vi "GrabAllData.vi"(3 "Type of scan":u16, 4 "All files":string[](array[string]), 5 "error in":errorcluster, 6 "lines per plane mod":i32, 7 "Synth App?":bool, 8 "save?":bool=TRUE, 9 "Xmit Ring":i16, 10 "Start Record":i32, 11 "Reverse ?":bool) -> ()   [LabVIEW 2022 SP3]
uses:
  ScanningControl/Motion Controllers/-MotionRoutines/MotionGlobals.vi
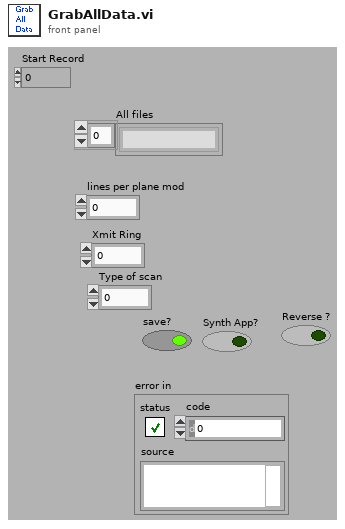
[diagram p1: front panel]
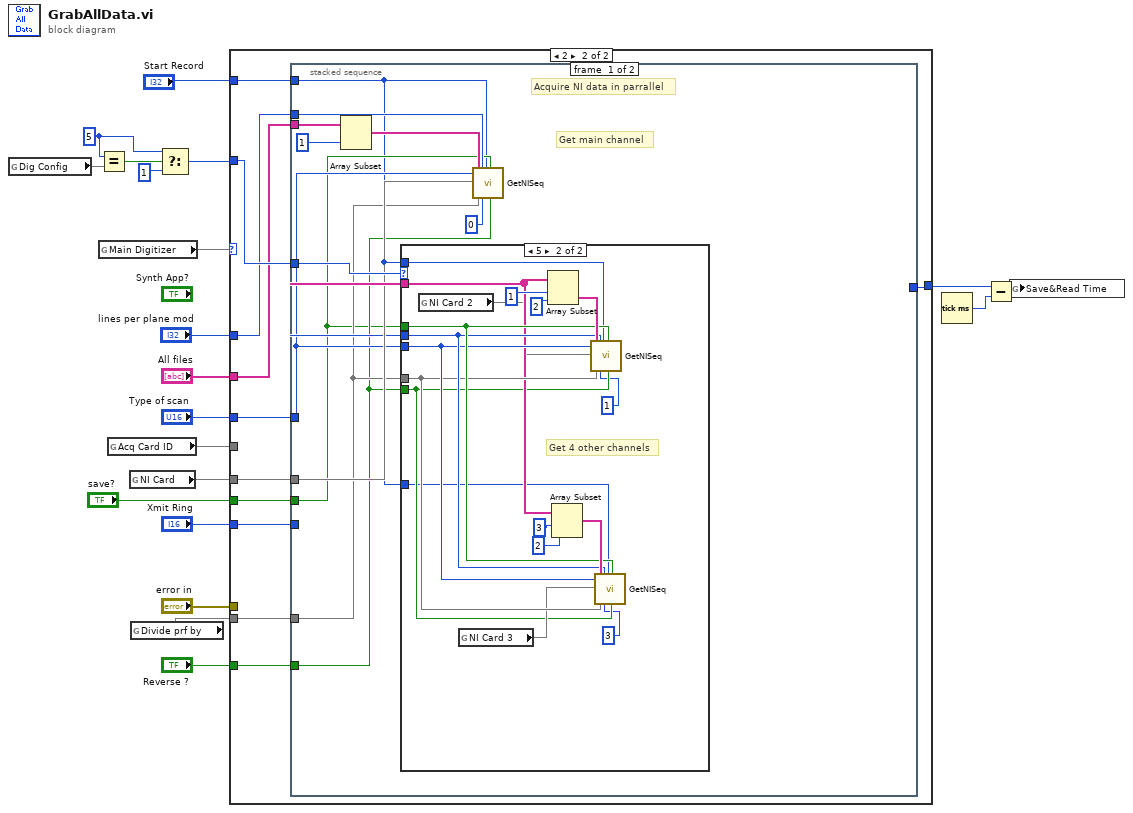
[diagram p0: block diagram]
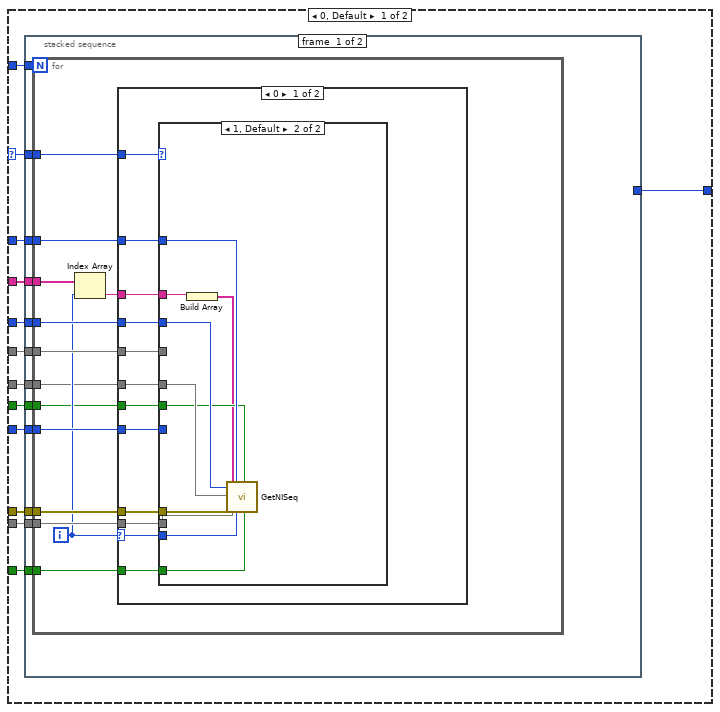
[diagram p2: hidden frame]
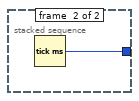
[diagram p5: hidden frame]
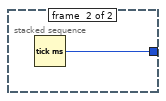
[diagram p7: hidden frame]
diagram:
  w20 = 5
  n1 = global read "MotionGlobals.vi" "Dig Config"() -> (w8)
  n2 = Equal?(x=w20, y=w8) -> (x = y?=w19:bool)
  n3 = global read "MotionGlobals.vi" "Main Digitizer"() -> (w5)
  n4 = global read "MotionGlobals.vi" "Acq Card ID"() -> (w10)
  n5 = global read "MotionGlobals.vi" "NI Card"() -> (w9)
  n6 = global read "MotionGlobals.vi" "Divide prf by"() -> (w7)
  n7 = Select(t=w20, s=w19, f=1) -> (s? t:f=w17:i32)
  n8 = case shown="2" w5 {
    selector: w5 -> [w22 _]
    tunnel: "All files" -> [w33 w91]
    tunnel: w17 -> [w32 w92]
    tunnel: "Xmit Ring" -> [w31 w87]
    tunnel: "Type of scan" -> [w30 w88]
    tunnel: "Reverse ?" -> [w29 w85]
    tunnel: "lines per plane mod" -> [w28 w89]
    tunnel: "error in" -> [w27 _]
    tunnel: w10 -> [w26 _]
    tunnel: w9 -> [w25 w90]
    tunnel: w7 -> [w24 w86]
    tunnel: "save?" -> [w23 w84]
    tunnel: [w21 w83] -> w4
    tunnel: "Start Record" -> [_ w82]
    frame 0, Default {
      n9 = stacked-sequence {
        tunnel: w33 -> [w45 _]
        tunnel: w32 -> [w44 _]
        tunnel: w31 -> [w43 _]
        tunnel: w30 -> [w42 _]
        tunnel: w29 -> [w41 _]
        tunnel: w28 -> [w40 _]
        tunnel: w27 -> [w39 _]
        tunnel: w26 -> [w38 _]
        tunnel: w25 -> [w37 _]
        tunnel: w24 -> [w36 _]
        tunnel: w23 -> [w35 _]
        tunnel: w22 -> [w34 _]
        tunnel: [_ w81] -> w21
        frame #0 {
          n10 = for {
            N: w44 -> [_]
            tunnel: w36 -> [w58]
            tunnel: w39 -> [w57]
            tunnel: w40 -> [w56]
            tunnel: w41 -> [w55]
            tunnel: w42 -> [w54]
            tunnel: w43 -> [w53]
            tunnel: w38 -> [w52]
            tunnel: w45 -> [w49]
            tunnel: w34 -> [w48]
            tunnel: w37 -> [w47]
            tunnel: w35 -> [w46]
            i -> [w50]
            n11 = Index Array(array=w49, index=w50) -> (element=w51:string)
            n12 = case shown="0" w50 {
              selector: w50 -> [w60 _]
              tunnel: w58 -> [w70 _]
              tunnel: w57 -> [w69 _]
              tunnel: w56 -> [w68 _]
              tunnel: w55 -> [w67 _]
              tunnel: w54 -> [w66 _]
              tunnel: w53 -> [w61 _]
              tunnel: w52 -> [w65 _]
              tunnel: w51 -> [w64 _]
              tunnel: w48 -> [w63 _]
              tunnel: w47 -> [w62 _]
              tunnel: w46 -> [w59 _]
              frame 0 {
                n13 = case shown="1, Default" w63 {
                  tunnel: w70 -> [_ w80]
                  tunnel: w69 -> [_ w79]
                  tunnel: w68 -> [_ w76]
                  tunnel: w67 -> [_ w75]
                  tunnel: w66 -> [_ w78]
                  tunnel: w61 -> [_ _]
                  tunnel: w65 -> [_ _]
                  tunnel: w64 -> [_ w73]
                  tunnel: w62 -> [_ w77]
                  tunnel: w60 -> [_ w71]
                  tunnel: w59 -> [_ w74]
                  frame 0 {
                    # "Get single channel Acqiris data"
                  }
                  frame 1, Default {
                    n14 = Build Array(w73) -> (w72:string[])
                    n15 = call "GetNISeq.vi"("Type of scan"=w78, "NI Card"=w77, "errorin"=w79, "File Array"=w72, "Divide prf by"=w80, "lines per plane"=w76, "Channel (0)"=w71, "save?"=w74, "Reverse?"=w75) -> ()  [unwired: 2 in, 17 out]
                  }
                }
              }
              frame 1, Default {
              }
            }
          }
        }
        frame #1 {
          n16 = Tick Count (ms)() -> (millisecond timer value=w81:u32)
        }
      }
    }
    frame 2 {
      n17 = stacked-sequence {
        tunnel: w92 -> [w103 _]
        tunnel: w91 -> [w102 _]
        tunnel: w90 -> [w101 _]
        tunnel: w89 -> [w100 _]
        tunnel: w88 -> [w99 _]
        tunnel: w87 -> [_ _]
        tunnel: w86 -> [w98 _]
        tunnel: w85 -> [w97 _]
        tunnel: w84 -> [w96 _]
        tunnel: [_ w123] -> w83
        tunnel: w82 -> [w94 _]
        frame #0 {
          # "Acquire NI data in parrallel"
          # "Get main channel"
          n18 = Array Subset(array=w102, length=1) -> (w104:string[])  [unwired: 1 in]
          n19 = case shown="5" w103 {
            tunnel: w102 -> [_ w114]
            tunnel: w97 -> [_ w109]
            tunnel: w98 -> [_ w115]
            tunnel: w96 -> [_ w118]
            tunnel: w100 -> [_ w117]
            tunnel: w99 -> [_ w116]
            tunnel: w94 -> [_ w108]
            tunnel: w94 -> [_ w107]
            frame 0, Default {
            }
            frame 5 {
              # "Get 4 other channels"
              n20 = global read "MotionGlobals.vi" "NI Card 2"() -> (w113)
              n21 = global read "MotionGlobals.vi" "NI Card 3"() -> (w112)
              n22 = Array Subset(array=w114, index=1, length=2) -> (w121:string[])
              n23 = Array Subset(array=w114, index=3, length=2) -> (w119:string[])
              n24 = call "GetNISeq.vi"("Type of scan"=w116, "NI Card"=w113, "File Array"=w121, "Divide prf by"=w115, "lines per plane"=w117, "Channel (0)"=1, "Start Record"=w107, "save?"=w118, "Reverse?"=w109) -> ()  [unwired: 2 in, 17 out]
              n25 = call "GetNISeq.vi"("Type of scan"=w116, "NI Card"=w112, "File Array"=w119, "Divide prf by"=w115, "lines per plane"=w117, "Channel (0)"=3, "Start Record"=w108, "save?"=w118, "Reverse?"=w109) -> ()  [unwired: 2 in, 17 out]
            }
          }
          n26 = call "GetNISeq.vi"("Type of scan"=w99, "NI Card"=w101, "File Array"=w104, "Divide prf by"=w98, "lines per plane"=w100, "Channel (0)"=0, "Start Record"=w94, "save?"=w96, "Reverse?"=w97) -> ()  [unwired: 2 in, 17 out]
        }
        frame #1 {
          n27 = Tick Count (ms)() -> (millisecond timer value=w123:u32)
        }
      }
    }
  }
  n28 = Tick Count (ms)() -> (millisecond timer value=w3:u32)
  n29 = Subtract(x=w4, y=w3) -> (x-y=w2:u32)
  n30 = global write "MotionGlobals.vi" "Save&Read Time"(w2) -> ()
